vi "Create New Build.vi"(7 "TargetItem Refnum":refnum<vi>, 8 "error in (no error)":errorcluster, 10 "Build specification name":string, 11 "Project Refnum":refnum<vi>) -> (0 "error out":errorcluster, 3 "SDIST out":refnum<class "NI_AB_API_SDIST.lvclass">)   [LabVIEW 2020, in "NI_AB_API_SDIST.lvclass"]
uses:
  <vilib>/AppBuilder/AB_API/SDIST/NI_AB_API_SDIST.lvclass
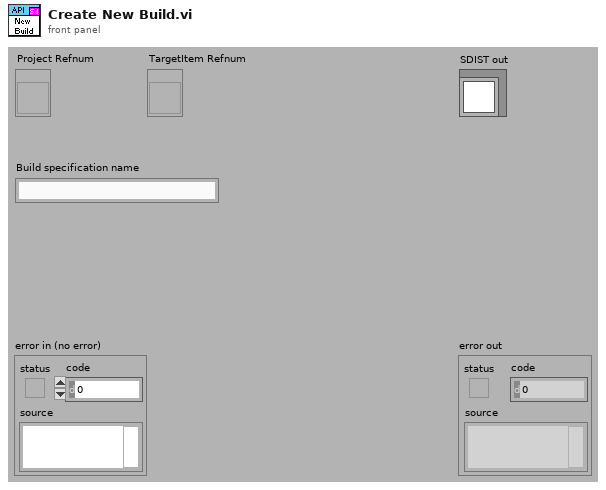
[diagram p1: front panel]
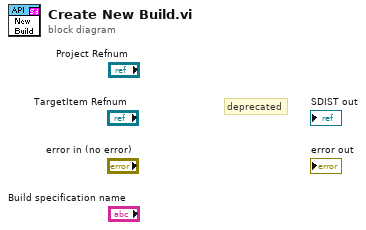
[diagram p0: block diagram]
diagram:
  # "deprecated"
